vi "UTILITY E-Time.vi"(6 "Set Start Time (s)":dbl format="%0.2f", 8 "error in (no error)":errorcluster, 9 "Reset":bool) -> (0 "error out":errorcluster, 1 "Elapsed Time (sec)":dbl format="%.2f", 4 "Time Since Last Run (sec)":dbl)   [LabVIEW 2016]
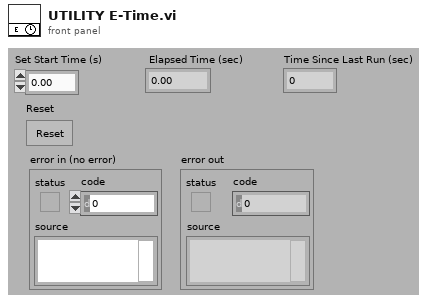
[diagram p1: front panel]
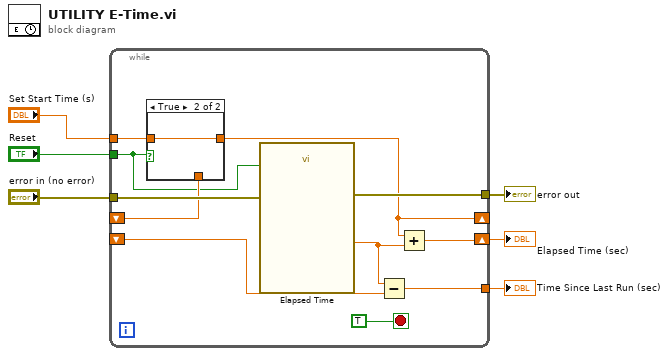
[diagram p0: block diagram]
diagram:
  n1 = while {
    tunnel: "Reset" -> [w7]
    tunnel: "error in (no error)" -> [w17]
    tunnel: [w16] -> w3
    shift-right: [w12] -> w6
    shift-left: _ -> [w15]
    tunnel: [w14] -> w2
    tunnel: "Set Start Time (s)" -> [w9]
    shift-right: [w10] -> _
    shift-left: _ -> [w8]
    stop <- TRUE stop-if-true
    n2 = case shown="True" w7 {
      tunnel: [w18 w19] -> w10
      tunnel: w9 -> [_ w19]
      tunnel: w8 -> [w18 _]
      frame False {
      }
      frame True {
      }
    }
    n3 = call "Elapsed Time"("Reset"=w7, "error in (no error)"=w17) -> ("Elapsed Time (s)"=w11:dbl, "error out"=w16:errorcluster)  [unwired: 10 in, 6 out]
    n4 = Subtract(x=w11, y=w15) -> (x-y=w14:dbl)
    n5 = Add(x=w10, y=w11) -> (x+y=w12:dbl)
  }
  "Elapsed Time (sec)" <- w6
  "error out" <- w3
  "Time Since Last Run (sec)" <- w2
